vi "Entry Source To Working.vi"(8 "Error In":errorcluster, 10 "Source File":path, 11 "VIChallenge Config":T1={"AWS Credentials"={"AWSAccessKeyId"="", "Secret Key"=""}, "AWS Account Number"="", "SQS Jobs"=refnum, "SQS Status"=refnum, "Source Dir"=path "", "Working Dir"=path "", "Output Dir"=path "", "Archive Dir"=path "", "job"={"job_id"="", "challenge_id"="", "user_id"="", "s3_source_bucket"="", "s3_source_directory"="", "s3_source_filename"="", "status_queue_name"="", "username"=""}, "Database Ref"=refnum, "Challenge Dir"=path "", "Challenges"=[]}) -> (0 "Error Out":errorcluster, 1 "Main VI Path":path, 3 "VIChallenge Config":T1)   [LabVIEW 2013, in "VIChallenge.lvlib"]
doc: "Clear Working Directory And Move Source File Into Working Directory (unzip if necissary)."
uses:
  VIChallenge.lvlib
  Type Defs/VIChallenge Config.ctl
  <vilib>/National Instruments/NI Amazon Web Services (AWS) Toolkit for LabVIEW/SQS/VI Source/AWS SQS Class/AWS_SQS.lvclass
  <vilib>/National Instruments/NI Amazon Web Services (AWS) Toolkit for LabVIEW/AWS Core Lib/VI Source/Canonicals/AWS_Core Canonical Credentials/Canonical Credentials.lvclass
  <vilib>/National Instruments/NI Amazon Web Services (AWS) Toolkit for LabVIEW/AWS Core Lib/VI Source/Canonicals/AWS_Core Canonical Required Parameters/Canonical Required Parameters.lvclass
  <vilib>/National Instruments/NI Amazon Web Services (AWS) Toolkit for LabVIEW/SQS/VI Source/Canonicals/Canonical CreateQueue/Canonical CreateQueue.lvclass
  <vilib>/National Instruments/NI Amazon Web Services (AWS) Toolkit for LabVIEW/SQS/VI Source/Canonicals/Canonical ListQueues/Canonical ListQueues.lvclass
  <vilib>/National Instruments/NI Amazon Web Services (AWS) Toolkit for LabVIEW/SQS/VI Source/Canonicals/Canonical AddPermission/Canonical AddPermission.lvclass
  <vilib>/National Instruments/NI Amazon Web Services (AWS) Toolkit for LabVIEW/SQS/VI Source/Canonicals/Canonical ChangeMessageVisibility/Canonical ChangeMessageVisibility.lvclass
  <vilib>/National Instruments/NI Amazon Web Services (AWS) Toolkit for LabVIEW/SQS/VI Source/Canonicals/Canonical ChangeMessageVisibilityBatch/Canonical ChangeMessageVisibilityBatch.lvclass
  <vilib>/National Instruments/NI Amazon Web Services (AWS) Toolkit for LabVIEW/SQS/VI Source/Canonicals/Canonical DeleteMessage/Canonical DeleteMessage.lvclass
  <vilib>/National Instruments/NI Amazon Web Services (AWS) Toolkit for LabVIEW/SQS/VI Source/Canonicals/Canonical DeleteMessageBatch/Canonical DeleteMessageBatch.lvclass
  <vilib>/National Instruments/NI Amazon Web Services (AWS) Toolkit for LabVIEW/SQS/VI Source/Canonicals/Canonical GetQueueAttributes/Canonical GetQueueAttributes.lvclass
  <vilib>/National Instruments/NI Amazon Web Services (AWS) Toolkit for LabVIEW/SQS/VI Source/Canonicals/Canonical GetQueueUrl/Canonical GetQueueUrl.lvclass
  <vilib>/National Instruments/NI Amazon Web Services (AWS) Toolkit for LabVIEW/SQS/VI Source/Canonicals/Canonical ReceiveMessage/Canonical ReceiveMessage.lvclass
  <vilib>/National Instruments/NI Amazon Web Services (AWS) Toolkit for LabVIEW/SQS/VI Source/Canonicals/Canonical RemovePermission/Canonical RemovePermission.lvclass
  <vilib>/National Instruments/NI Amazon Web Services (AWS) Toolkit for LabVIEW/SQS/VI Source/Canonicals/Canonical SendMessage/Canonical SendMessage.lvclass
  <vilib>/National Instruments/NI Amazon Web Services (AWS) Toolkit for LabVIEW/SQS/VI Source/Canonicals/Canonical SendMessageBatch/Canonical SendMessageBatch.lvclass
  <vilib>/National Instruments/NI Amazon Web Services (AWS) Toolkit for LabVIEW/SQS/VI Source/Canonicals/Canonical SetQueueAttributes/Canonical SetQueueAttributes.lvclass
  <vilib>/National Instruments/NI Amazon Web Services (AWS) Toolkit for LabVIEW/AWS Core Lib/VI Source/Typedefs/AWS_AWS Credentials.ctl
  Type Defs/JSON_job.ctl
  <vilib>/addons/database/Connection.llb/Conn ObjectReference.ctl
  Type Defs/Challenge.ctl
  <vilib>/zip/NI_Unzip.lvlib
  <vilib>/LabVIEW Hacker/LVH-Toolbox/Common/LVH-Common.lvlib
  <vilib>/National Instruments/NI Amazon Web Services (AWS) Toolkit for LabVIEW/AWS Core Lib/VI Source/AWS_Core.lvlib
  <vilib>/addons/database/NI_Database_API.lvlib
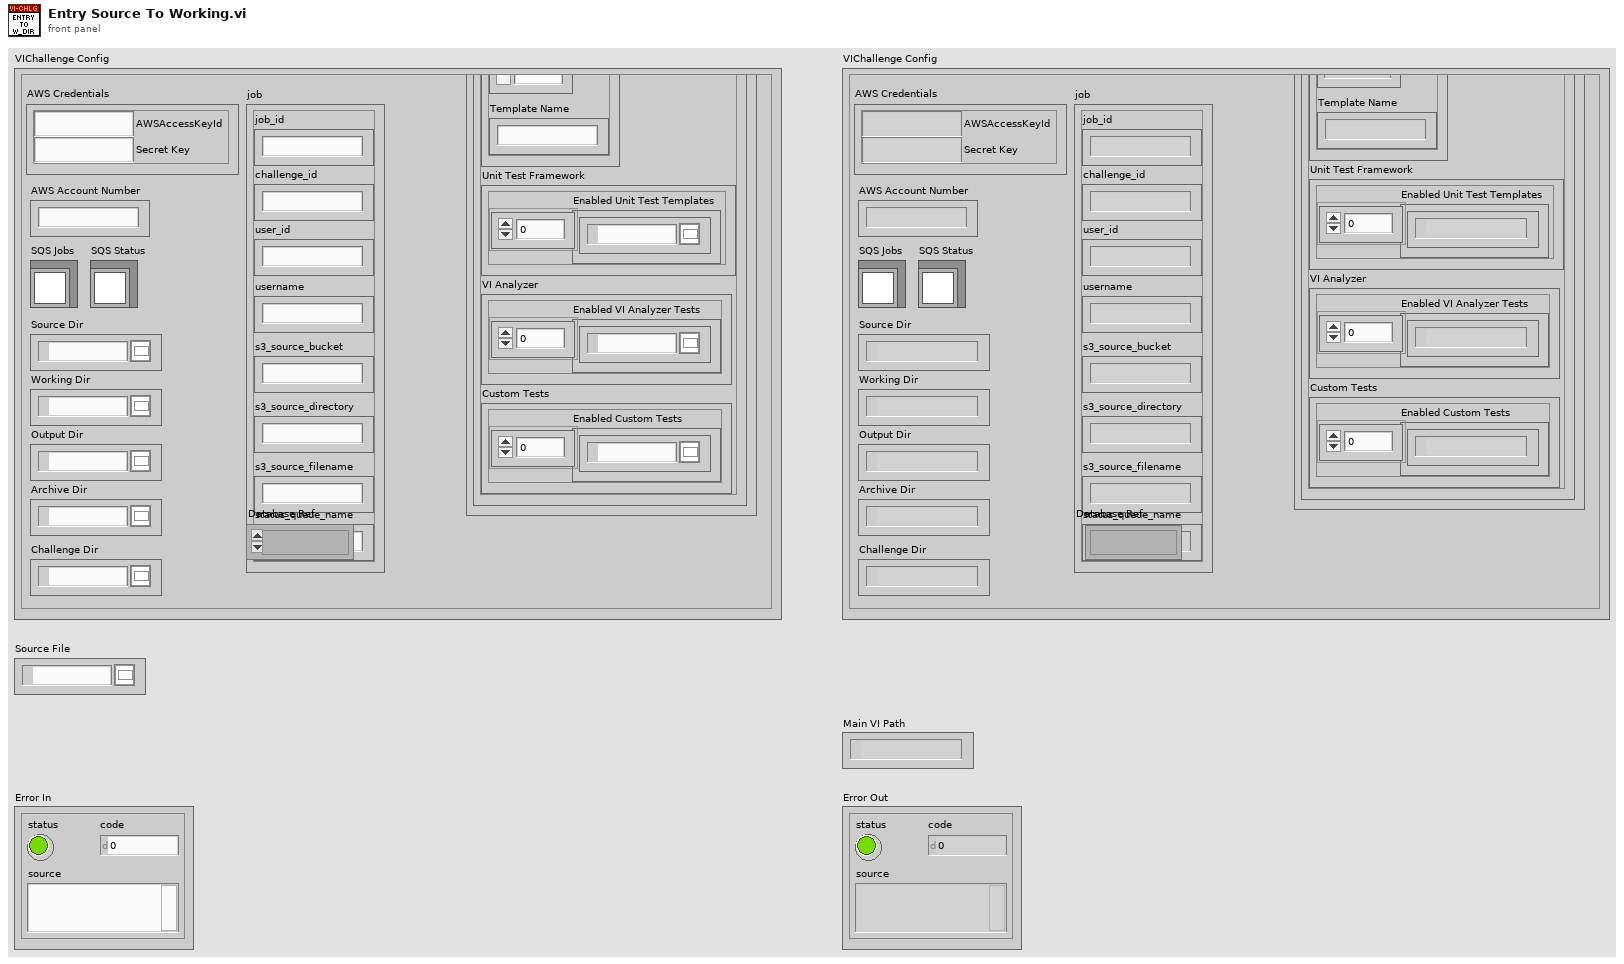
[diagram p1: front panel]
types:
  T1 = typedef "VIChallenge.lvlib/VIChallenge Config.ctl" = cluster{"AWS Credentials":T2, "AWS Account Number":string, "SQS Jobs":refnum<class "AWS_SQS.lvclass">, "SQS Status":refnum<class "AWS_SQS.lvclass">, "Source Dir":path, "Working Dir":path, "Output Dir":path, "Archive Dir":path, "job":T3, "Database Ref":T4, "Challenge Dir":path, "Challenges":T5[]}
  T2 = typedef "AWS_Core.lvlib/AWS_AWS Credentials.ctl" = cluster{"AWSAccessKeyId":string, "Secret Key":string}
  T3 = typedef "VIChallenge.lvlib/JSON_job.ctl" = cluster{"job_id":string, "challenge_id":string, "user_id":string, "s3_source_bucket":string, "s3_source_directory":string, "s3_source_filename":string, "status_queue_name":string, "username":string}
  T4 = typedef "NI_Database_API.lvlib/Conn ObjectReference.ctl" = refnum<k1>
  T5 = typedef "VIChallenge.lvlib/Challenge.ctl" = cluster{"General":cluster{"Challenge Id":i32, "Template Name":string}, "Unit Test Framework":cluster{"Enabled Unit Test Templates":path[]}, "VI Analyzer":cluster{"Enabled VI Analyzer Tests":path[]}, "Custom Tests":cluster{"Enabled Custom Tests":path[]}}
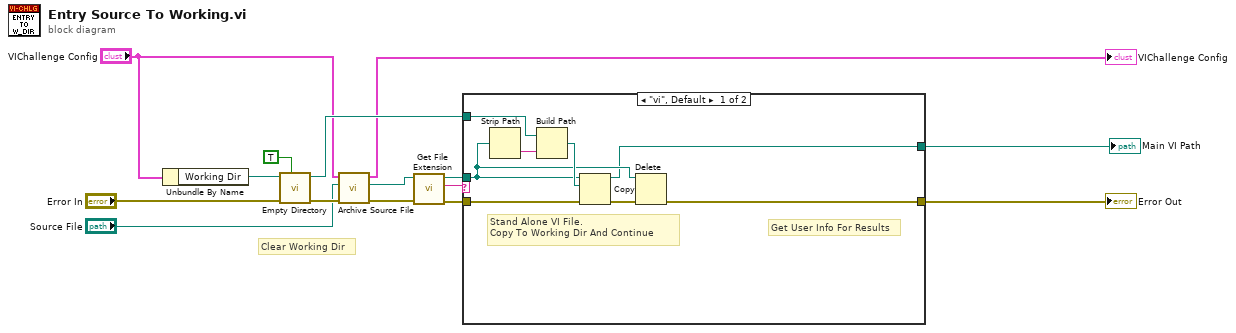
[diagram p0: block diagram]
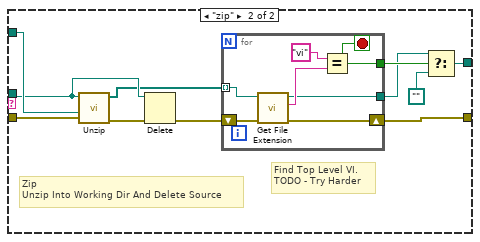
[diagram p2: hidden frame]
diagram:
  # "Clear Working Dir"
  n1 = Unbundle By Name("VIChallenge Config") -> ("Working Dir"=w9:path)
  n2 = call <vilib>:"Empty Directory.vi"("Delete Files Without Prompt? (F)"=TRUE, "Error In"="Error In", "Directory"=w9) -> ("Error Out"=w8:errorcluster, "Duplicate Path"=w15:path)  [unwired: 6 in, 1 out]
  n3 = call "Archive Source File.vi"("Error In"=w8, "Source File"="Source File", "VIChallenge Config"="VIChallenge Config") -> ("Error Out"=w5:errorcluster, "Dup Source File"=w6:path, "VIChallenge Config"=→"VIChallenge Config":T1)  [unwired: 6 in]
  n4 = call <vilib>:"Get File Extension.vi"("error in (no error)"=w5, "file"=w6) -> ("error out"=w12:errorcluster, "lowercase file extension"=w10:string, "dup file"=w11:path)  [unwired: 6 in, 1 out]
  n5 = case shown="\"vi\", Default" w10 {
    tunnel: w11 -> [w19 w31]
    tunnel: w15 -> [w22 w33]
    tunnel: w12 -> [w20 w34]
    tunnel: [w16 w29] -> w1
    tunnel: [w17 w27] -> w2
    frame "vi", Default {
      # "Get User Info For Results"
      # "Stand Alone VI File.  \nCopy To Working Dir And Continue"
      n6 = Strip Path(path=w19) -> (name=w23:string)  [unwired: 1 out]
      n7 = Build Path(base path=w22, name or relative path=w23) -> (appended path=w21:path)
      n8 = Copy(8:w20, 10:w21, 11:w19) -> (0:w18:errorcluster, 3:w17:path)  [unwired: 2 in, 1 out]
      n9 = Delete(path (use dialog)=w19, error in=w18) -> (error out=w16:errorcluster)  [unwired: 3 in, 2 out]
    }
    frame "zip" {
      # "Find Top Level VI. \nTODO - Try Harder"
      # "Zip\nUnzip Into Working Dir And Delete Source"
      n10 = call <vilib>:"Unzip.vi"("error in (no error)"=w34, "Target directory (same as Zip file if empty)"=w33, "Zip file"=w31) -> ("error out"=w32:errorcluster, "Unzipped files"=w30:path[])  [unwired: 6 in, 1 out]
      n11 = Delete(path (use dialog)=w31, error in=w32) -> (error out=w28:errorcluster)  [unwired: 3 in, 2 out]
      n12 = for {
        tunnel: w30 -> [w41] mode=indexing
        tunnel: [w36] -> w26
        tunnel: [w35] -> w25
        shift-right: [w39] -> w29
        shift-left: w28 -> [w40]
        stop <- w36 stop-if-true
        n13 = call <vilib>:"Get File Extension.vi"("error in (no error)"=w40, "file"=w41) -> ("error out"=w39:errorcluster, "lowercase file extension"=w38:string, "dup file"=w35:path)  [unwired: 6 in, 1 out]
        n14 = Equal?(x="vi", y=w38) -> (x = y?=w36:bool)
      }
      n15 = Select(t=w25, s=w26, f=path "") -> (s? t:f=w27:path)
    }
  }
  "Error Out" <- w1
  "Main VI Path" <- w2
